vi "TestAsylumMethods.vi"(8 "error in (no error)":errorcluster) -> (0 "error out":errorcluster)   [LabVIEW 2016]
uses:
  <vilib>/addons/_JKI Toolkits/Caraya/classes/Test/Test.lvclass
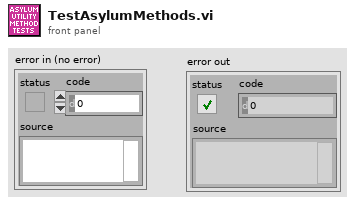
[diagram p1: front panel]
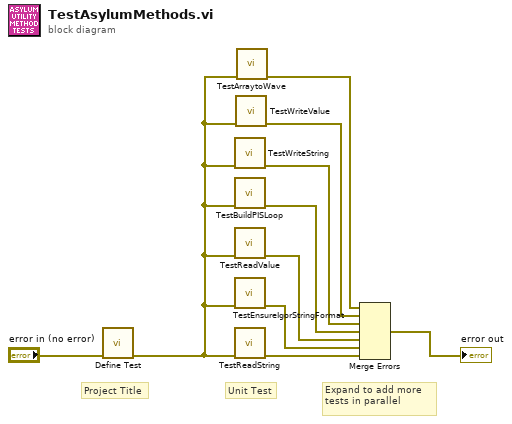
[diagram p0: block diagram]
diagram:
  # "Expand to add more tests in parallel"
  # "Unit Test"
  # "Project Title"
  n1 = call <vilib>:"Define Test.vi"("error in (no error)"="error in (no error)") -> ("error out"=w2:errorcluster)  [unwired: 10 in]
  n2 = call "TestWriteString.vi"("error in (no error)"=w2) -> ("error out"=w4:errorcluster)  [unwired: 10 in]
  n3 = call "TestBuildPISLoop.vi"("error in (no error)"=w2) -> ("error out"=w5:errorcluster)  [unwired: 10 in]
  n4 = call "TestReadValue.vi"("error in (no error)"=w2) -> ("error out"=w6:errorcluster)  [unwired: 10 in]
  n5 = call "TestEnsureIgorStringFormat.vi"("error in (no error)"=w2) -> ("error out"=w7:errorcluster)  [unwired: 10 in]
  n6 = call "TestReadString.vi"("error in (no error)"=w2) -> ("error out"=w8:errorcluster)  [unwired: 10 in]
  n7 = call "TestWriteValue.vi"("error in (no error)"=w2) -> ("error out"=w3:errorcluster)  [unwired: 10 in]
  n8 = call "TestArraytoWave.vi"("error in (no error)"=w2) -> ("error out"=w1:errorcluster)  [unwired: 10 in]
  n9 = Merge Errors(w1, w3, w4, w5, w6, w7, w8) -> (→"error out":errorcluster)
